vi "MeasureKeithleyandSend.vi"(0 "Keithley Visa name":refnum<visa-resource-name>, 1 "QueueCluster":T2, 5 "Node In":string, 7 "MainMsg":T3, 9 "GUIMsg":T4, 11 "error in (no error)":errorcluster, 12 "MeasureFunction":T1(ring)) -> (15 "error out":errorcluster)   [LabVIEW 2017]
uses:
  CTRLS/GUIMsg.ctl
  MainMsg.ctl
  CTRLS/EventCluster.ctl
  CTRLS/ListenMsg.ctl
  CTRLS/MainCluster.ctl
  CTRLS/DAQCluster.ctl
  DaqMsg.ctl
  CTRLS/GUICluster.ctl
  Keithley 2600 Series/Public/Channel.ctl
  <vilib>/express/express arith-compare/Formula/XNode/ExpressFormulaBlockNode.xnode
  Keithley 2600 Series/Keithley 2600 Series.lvlib
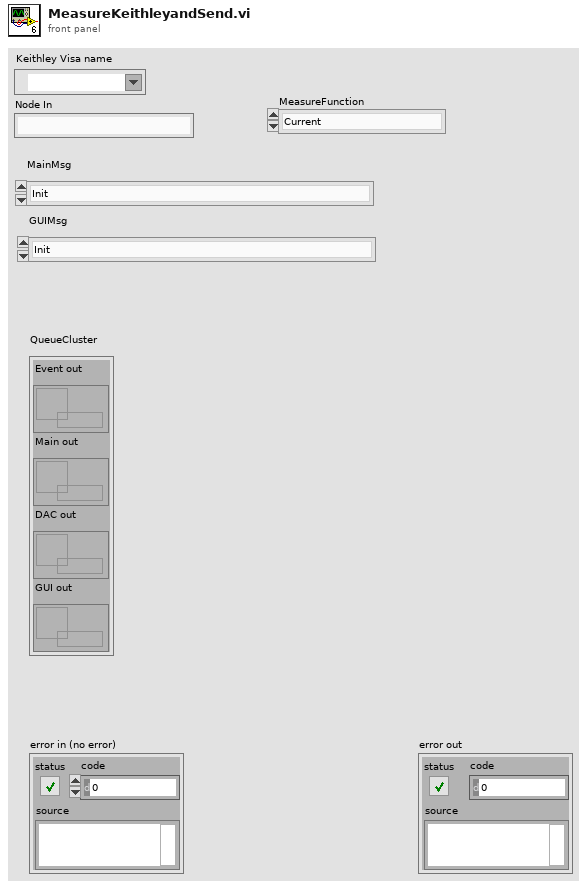
[diagram p1: front panel]
types:
  T1 = enum32{"Current", "Voltage", "IV", "Resistance", "Power"}
  T2 = cluster{"Event out":refnum<queue>, "Main out":refnum<queue>, "DAC out":refnum<queue>, "GUI out":refnum<queue>}
  T3 = typedef "MainMsg.ctl" = enum16{"Init", "Halt", "MonitorState", "SaveState", "Filename", "AirFlow", "WaterFlow", "AirPress", "WaterPress", "WaterTemp", "NozzleForce", "SaveAll", "Error", "Supervisor"}
  T4 = typedef "GUIMsg.ctl" = enum16{"Init", "Halt", "WaterFlow", "AirFlow", "WaterPress", "AirPress", "WaterTemp", "NozzleForce", "SaveState", "MonState"}
  T5 = typedef "GUICluster.ctl" = cluster{"GUIMsg":T4, "GUINum":dbl, "GUIStr":string}
  T6 = typedef "MainCluster.ctl" = cluster{"MainMsg":T3, "MainNum":dbl, "MainStr":string}
  T7 = typedef "Keithley 2600 Series.lvlib/Channel.ctl" = enum32{"Channel A", "Channel B"}
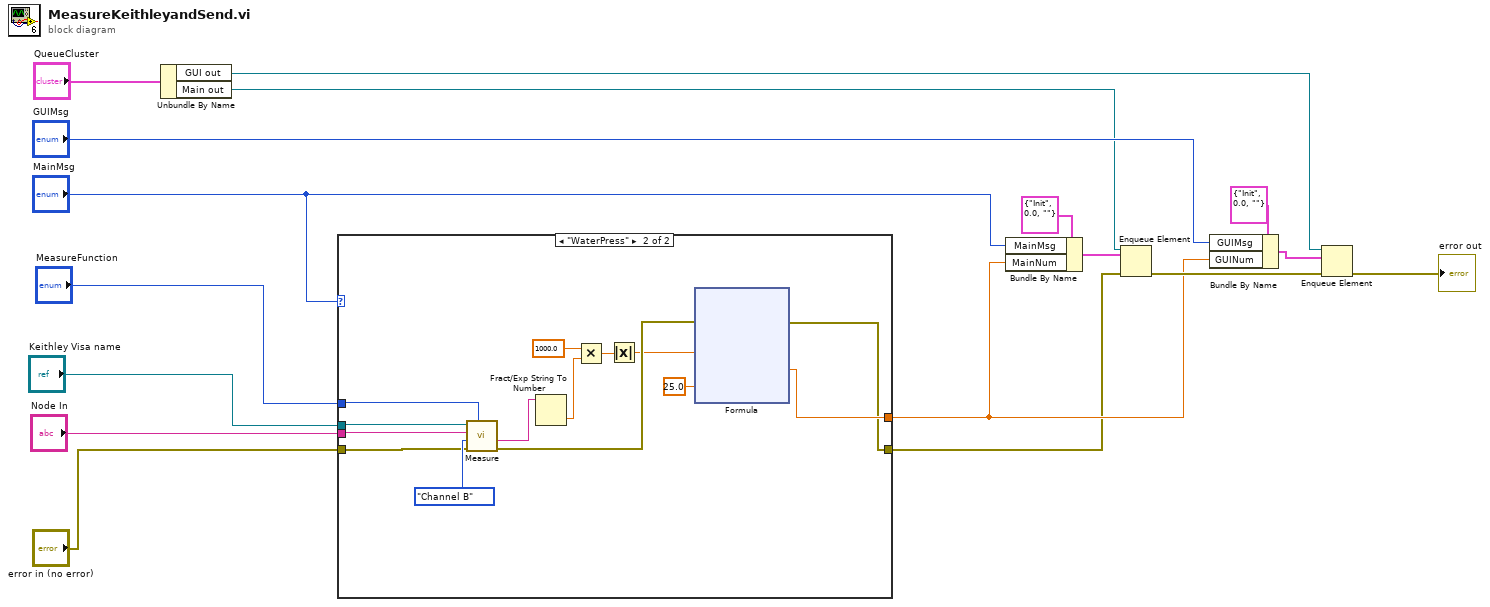
[diagram p0: block diagram]
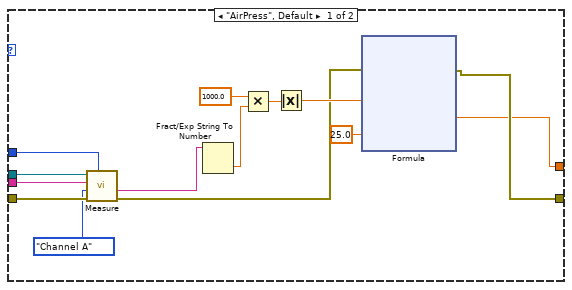
[diagram p2: hidden frame]
diagram:
  n1 = Unbundle By Name("QueueCluster") -> ("GUI out"=w13:refnum<queue>, "Main out"=w9:refnum<queue>)
  n2 = case shown="\"WaterPress\"" "MainMsg" {
    tunnel: "error in (no error)" -> [w31 w50]
    tunnel: "Node In" -> [w30 w51]
    tunnel: "Keithley Visa name" -> [w29 w52]
    tunnel: "MeasureFunction" -> [w27 w53]
    tunnel: [w18 w49] -> w2
    tunnel: [w19 w47] -> w1
    frame "AirPress", Default {
      n3 = call "Measure.vi"("Function (Current)"=w27, "error in (no error)"=w31, "Channel (Channel A)"=Channel."Channel A", "Node In"=w30, "VISA resource name"=w29) -> ("error out"=w20:errorcluster, "Output"=w21:string)  [unwired: 2 in, 3 out]
      n4 = Fract/Exp String To Number(string=w21) -> (number=w24:dbl)  [unwired: 3 in, 1 out]
      n5 = Multiply(x=1000.0, y=w24) -> (x*y=w23:dbl)
      n6 = Absolute Value(x=w23) -> (abs(x)=w26:dbl)
      n7 = xnode "Formula"("Current"=w26, "MaxVal"=25.0, "error in (no error)"=w20) -> ("Result"=w18:dbl, "error out"=w19:errorcluster)
    }
    frame "WaterPress" {
      n8 = call "Measure.vi"("Function (Current)"=w53, "error in (no error)"=w50, "Channel (Channel A)"=Channel."Channel B", "Node In"=w51, "VISA resource name"=w52) -> ("error out"=w48:errorcluster, "Output"=w54:string)  [unwired: 2 in, 3 out]
      n9 = Fract/Exp String To Number(string=w54) -> (number=w44:dbl)  [unwired: 3 in, 1 out]
      n10 = Multiply(x=1000.0, y=w44) -> (x*y=w43:dbl)
      n11 = Absolute Value(x=w43) -> (abs(x)=w46:dbl)
      n12 = xnode "Formula"("Current"=w46, "MaxVal"=25.0, "error in (no error)"=w48) -> ("Result"=w49:dbl, "error out"=w47:errorcluster)
    }
  }
  n13 = Bundle By Name(cluster=T6 {"MainMsg"=enum."Init", "MainNum"=0.0, "MainStr"=""} ("element"), "MainMsg"="MainMsg", "MainNum"=w2) -> (w11:T6)
  n14 = Enqueue Element(queue=w9, element=w11, error in (no error)=w1) -> (error out=w12:errorcluster)  [unwired: 1 in, 2 out]
  n15 = Bundle By Name(cluster=T5 {"GUIMsg"=enum."Init", "GUINum"=0.0, "GUIStr"=""} ("element"), "GUIMsg"="GUIMsg", "GUINum"=w2) -> (w15:T5)
  n16 = Enqueue Element(queue=w13, element=w15, error in (no error)=w12) -> (error out=→"error out":errorcluster)  [unwired: 1 in, 2 out]
